vi "SP Save Formatting.vi"(4 "s parameter formatting":T1 {"Plots"."Ch 2"."Reference" format="%#.2g"; "Plots"."Ch 2"."Display Data" items=["Data", "Memory", "Data/Memory"]; "Plots"."Ch 2"."Format" items=["Log Mag", "Phase", "Expanded Phase", "Delay", "Smith", "Polar", "Lin Mag", "SWR", "Loss", "Real", "Imaginary"]; "Plots"."Ch 2"."Scale" min=0.001 step=1.0 format="%#.2g"; "Plots"."Ch 2"."Position" min=0.0 max=10.0; "Plots"."Ch 1"."Reference" format="%#.2g"; "Plots"."Ch 1"."Display Data" items=["Data", "Memory", "Data/Memory"]; "Plots"."Ch 1"."Format" items=["Log Mag", "Phase", "Expanded Phase", "Delay", "Smith", "Polar", "Lin Mag", "SWR", "Loss", "Real", "Imaginary"]; "Plots"."Ch 1"."Scale" min=0.001 step=1.0 format="%#.2g"; "Plots"."Ch 1"."Position" min=0.0 max=10.0}, 5 "error in (no error)":errorcluster, 6 "Cachefile Path (empty)":path, 7 "Object Hierarchy (empty)":string[](array[string]), 8 "tdms file Ref":refnum<k34>) -> (0 "error out":errorcluster, 2 "new Object Hierarchy":string[](array[string]), 3 "dup tdms file Ref":refnum<k34>)   [LabVIEW 2011]
uses:
  server/dd/lib/Report Templates/Template TDM/enumObjectTypes.ctl
  server/dd/lib/Report Templates/Template TDM/enumColor.ctl
  server/dd/lib/Report Templates/Template TDM/enumQueryResultTypes.ctl
  server/dd/lib/Report Templates/Template TDM/enumConditionType.ctl
  server/dd/lib/Report Templates/Template TDM/enumConditionOperator.ctl
  server/dd/lib/Report Templates/Template TDM/objQuery.ctl
  server/dd/lib/Report Templates/Template TDM/enumQueryKeyClass.ctl
  server/dd/lib/Report Templates/Template TDM/enumLineTypes.ctl
  server/dd/lib/Report Templates/Template TDM/enumLineWidths.ctl
  server/dd/lib/Report Templates/Template TDM/enumMarkerTypes.ctl
  TypeDefs/SP Trace.ctl
  TypeDefs/SP Trace Types.ctl
  TypeDefs/SP Frequency Units.ctl
  server/dd/lib/Report Templates/Template TDM/objPlacement.ctl
  TypeDefs/SP Trace Orientation.ctl
  server/dd/lib/Report Templates/Template TDM/enumSummaryOperator.ctl
  TypeDefs/SP Plot Channel.ctl
  TypeDefs/SP Plot Orientation.ctl
  TypeDefs/SP Plot.ctl
  TypeDefs/SP Display Format.ctl
  TypeDefs/SP Display Data.ctl
  TypeDefs/SP Display Trace Controls.ctl
  TypeDefs/SP Formatting.ctl
panel:
  # "Div"
  # "Div"
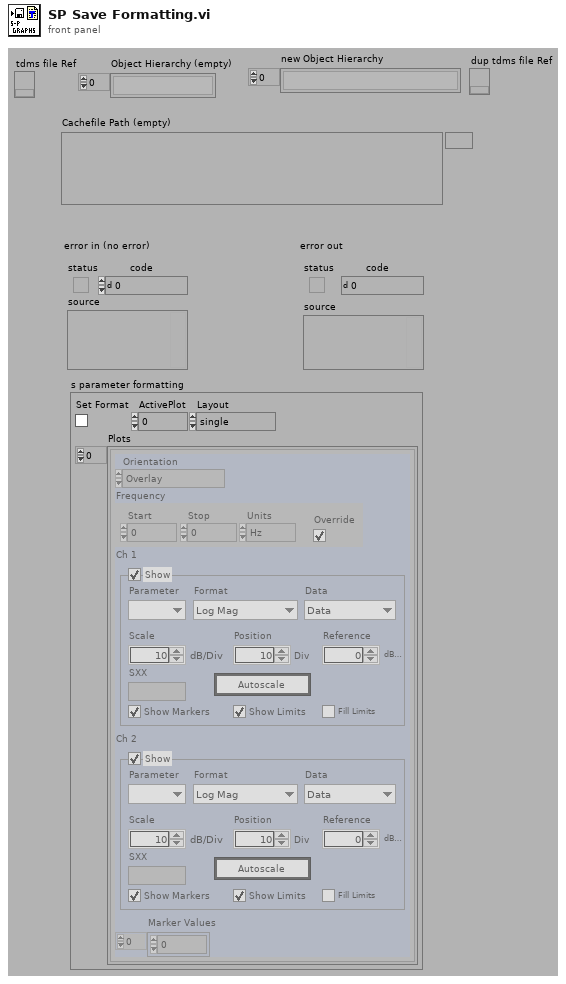
[diagram p1: front panel]
types:
  T1 = typedef "SP Formatting.ctl" = cluster{"Set Format":bool, "Layout":T2, "ActivePlot":i32, "Plots":T3[]}
  T2 = typedef "SP Plot Orientation.ctl" = enum32{"single", "dual", "quad"}
  T3 = typedef "SP Plot.ctl" = cluster{"Orientation":T4, "Ch 1":T5, "Ch 2":T5, "Frequency":cluster{"Start":dbl, "Stop":dbl, "Units":T8, "Override":bool}, "Marker Values":dbl[]}
  T4 = typedef "SP Trace Orientation.ctl" = enum32{"Overlay", "Split"}
  T5 = typedef "SP Display Trace Controls.ctl" = cluster{"Trace On":bool, "Measure":i32, "Format":T6, "Autoscale":bool, "Reference":dbl, "\nRefUnit":string, "Position":dbl, "Scale":dbl, "ScaleUnit":string, "LimitOn":bool, "LimitFill":bool, "Display Data":T7, "Show Markers":bool, "SXX":string}
  T6 = typedef "SP Display Format.ctl" = i32
  T7 = typedef "SP Display Data.ctl" = u16
  T8 = typedef "SP Frequency Units.ctl" = enum16{"Hz", "kHz", "MHz", "GHz", "Points"}
  T9 = enum16{"open", "open or create", "create or replace", "create", "open (read-only)"}
  T10 = typedef "objPlacement.ctl" = cluster{"XPos":dbl, "YPos":dbl, "Width":dbl, "Height":dbl}
  T11 = typedef "enumObjectTypes.ctl" = enum16{"container", "graphics", "text", "picture", "qobject", "sparameterplot", "sparametertrace"}
  T12 = typedef "objQuery.ctl" = cluster{"ResultType":T13, "KeyName":string, "KeyClass":T14, "NoResults":string, "IncludeUnit":bool, "ResultOffset":i32, "SummaryChannel":string, "SummaryFormat":string, "SummaryOperator":T15, "SummaryLimit":i32, "Conditions":cluster{"Type":T16, "Property":string, "Operator":T17, "Value":string}[]}
  T13 = typedef "enumQueryResultTypes.ctl" = enum16{"PropertyValue", "Scalar", "Vector", "Summary"}
  T14 = typedef "enumQueryKeyClass.ctl" = enum16{"File", "Run", "Channel"}
  T15 = typedef "enumSummaryOperator.ctl" = enum16{"avg", "min", "max", "rng", "sum"}
  T16 = typedef "enumConditionType.ctl" = enum16{"eSearchFile", "eSearchChannelGroup", "eSearchChannel"}
  T17 = typedef "enumConditionOperator.ctl" = enum16{"="}
  T18 = typedef "SP Plot Channel.ctl" = cluster{"ChIndex":i32, "Sxx":string, "Format":string, "Autoscale":bool, "Scale":dbl, "RefValue":dbl, "RefPos":dbl, "Fstart":dbl, "Fstop":dbl, "Funit":T8, "Color":T19, "DataQuery":string, "Markers":bool}
  T19 = typedef "enumColor.ctl" = enum16{"black", "red", "green", "blue", "violet", "turquoise", "grey", "yell", "dark red", "dark green", "dark blue", "dark violet", "dark turquoise", "dark grey", "dark yellow", "white", "other colors", "no color"}
  T20 = typedef "SP Trace.ctl" = cluster{"PlotName":string, "TraceSxx":string, "TraceType":T21, "Class":string, "Color":T19, "LineType":T22, "LineWidth":T23, "MarkerType":T24, "MarkerColor":T19, "MarkerSize":dbl}
  T21 = typedef "SP Trace Types.ctl" = enum16{"hidden", "data", "upper limit", "lower limit", "failures", "memory"}
  T22 = typedef "enumLineTypes.ctl" = enum16{"solid", "dash&dott", "dashed 1", "dashed 2", "dotted"}
  T23 = typedef "enumLineWidths.ctl" = enum16{"min", "0.25", "0.35", "0.5", "0.7", "1.0", "1.4", "2.0", "2.8", "4.0", "5.6", "8.0", "11.2", "16.0", "22.4", "32.0"}
  T24 = typedef "enumMarkerTypes.ctl" = enum16{"none", "square", "rhomb", "triangle", "cross", "asterisk", "short dash", "long dash", "plus", "circle"}
  T25 = cluster{"Start":dbl, "Stop":dbl, "Units":T8, "Override":bool}
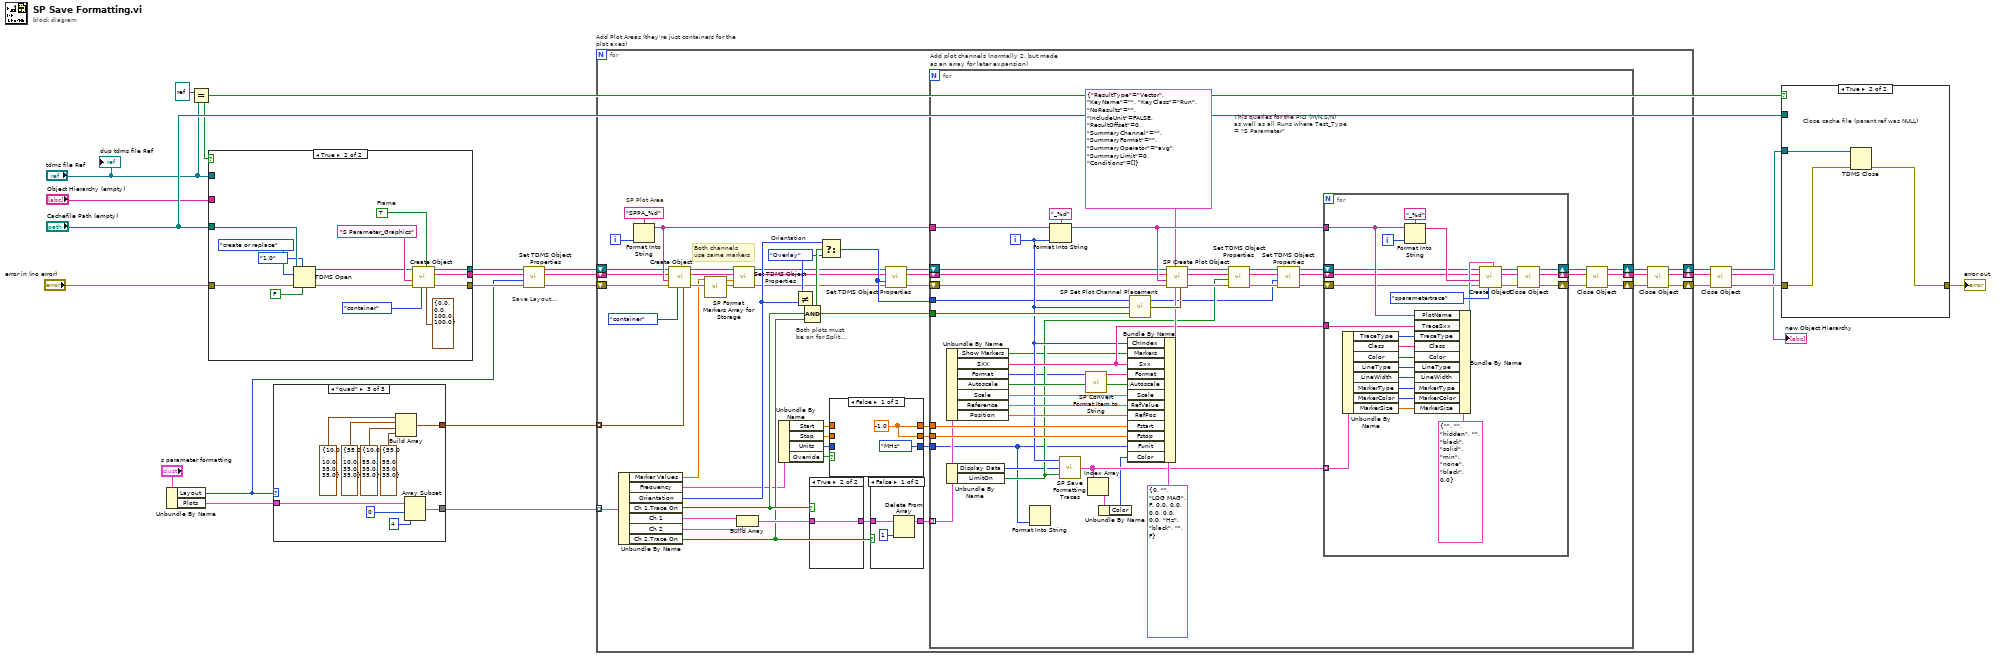
[diagram p0: block diagram]
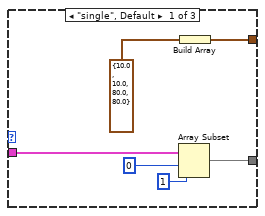
[diagram p2: hidden frame]
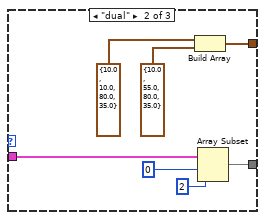
[diagram p3: hidden frame]
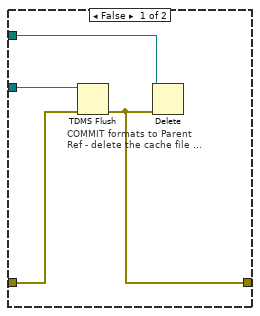
[diagram p4: hidden frame]
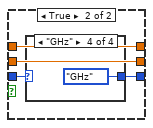
[diagram p6: hidden frame]
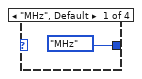
[diagram p7: hidden frame]
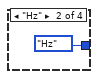
[diagram p8: hidden frame]
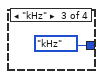
[diagram p9: hidden frame]
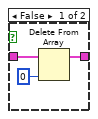
[diagram p11: hidden frame]
diagram:
  # "Save Layout..."
  n1 = Unbundle By Name("s parameter formatting") -> ("Layout"=w17:T2, "Plots"=w22:T3[])
  n2 = Equal?(x=refnum<k34> refnum ("tdms file Ref"), y="tdms file Ref") -> (x = y?=w3:bool)
  n3 = case shown="True" w3 {
    tunnel: "error in (no error)" -> [w27 w36]
    tunnel: "tdms file Ref" -> [w26 _]
    tunnel: [w27 w37] -> w20
    tunnel: "Cachefile Path (empty)" -> [_ w34]
    tunnel: [w25 w31] -> w14
    tunnel: [w26 w30] -> w16
    tunnel: "Object Hierarchy (empty)" -> [w25 _]
    frame False {
    }
    frame True {
      w39 = TRUE  # Frame
      n4 = TDMS Open(6:FALSE ("disable buffering (T)"), 7:enum16{"1.0", "2.0"}."1.0" ("file format version (2.0)"), 8:w36, 10:T9."create or replace" ("operation (0:open)"), 11:w34) -> (0:w35:errorcluster, 3:w32:refnum<k34>)  [unwired: 1 in]
      n5 = call "Create Object.vi"("Object Placement"=T10 {"XPos"=0.0, "YPos"=0.0, "Width"=100.0, "Height"=100.0} ("Placement"), "Properties"=w39, "Object Type (container)"=enumObjectTypes."container", "error in (no error)"=w35, "Object Name (\"\")"="S Parameter_Graphics", "tdms file Ref"=w32) -> ("error out"=w37:errorcluster, "new Object Hierarchy"=w31:string[], "dup tdms file Ref"=w30:refnum<k34>)  [unwired: 2 in, 1 out]
    }
  }
  n6 = case shown="\"quad\"" w17 {
    tunnel: [w46 w52 w62] -> w21
    tunnel: w22 -> [w45 w49 w58]
    tunnel: [w42 w48 w57] -> w1
    frame "single", Default {
      n7 = Array Subset(array=w45, index=0, length=1) -> (w42:T3[])
      n8 = Build Array(T10 {"XPos"=10.0, "YPos"=10.0, "Width"=80.0, "Height"=80.0} ("Placement")) -> (w46:T10[])
    }
    frame "dual" {
      n9 = Build Array(T10 {"XPos"=10.0, "YPos"=10.0, "Width"=80.0, "Height"=35.0} ("Placement"), T10 {"XPos"=10.0, "YPos"=55.0, "Width"=80.0, "Height"=35.0} ("Placement")) -> (w52:T10[])
      n10 = Array Subset(array=w49, index=0, length=2) -> (w48:T3[])
    }
    frame "quad" {
      n11 = Build Array(T10 {"XPos"=10.0, "YPos"=10.0, "Width"=35.0, "Height"=35.0} ("Placement"), T10 {"XPos"=55.0, "YPos"=10.0, "Width"=35.0, "Height"=35.0} ("Placement"), T10 {"XPos"=10.0, "YPos"=55.0, "Width"=35.0, "Height"=35.0} ("Placement"), T10 {"XPos"=55.0, "YPos"=55.0, "Width"=35.0, "Height"=35.0} ("Placement")) -> (w62:T10[])
      n12 = Array Subset(array=w58, index=0, length=4) -> (w57:T3[])
    }
  }
  n13 = call "Set TDMS Object Properties.vi"("error in (no error)"=w20, "Cluster or Control"=w17, "Object Hierarchy (empty)"=w14, "tdms file Ref"=w16) -> ("error out"=w7:errorcluster, "dup Object Hierarchy"=w13:string[], "dup tdms file Ref"=w8:refnum<k34>)  [unwired: 1 out]
  n14 = for "Add Plot Areas (they're just containers for the plot axes)" {
    tunnel: w21 -> [w105] mode=indexing
    tunnel: w1 -> [w104] mode=indexing
    shift-right: [w84] -> w10
    shift-left: w13 -> [w82]
    shift-right: [w78] -> w5
    shift-left: w8 -> [w80]
    shift-right: [w79] -> w6
    shift-left: w7 -> [w81]
    i -> [w107]
    w88 = SP_Trace_Orientation."Overlay"  # Orientation
    # "Both channels\nuse same markers"
    # "Both plots must\nbe on for Split..."
    # "SP Plot Area"
    n15 = Unbundle By Name(w104) -> ("Marker Values"=w66:dbl[], "Frequency"=w87:T25, "Orientation"=w89:T4, "Ch 1.Trace On"=w93:bool, "Ch 1"=w65:T5, "Ch 2"=w64:T5, "Ch 2.Trace On"=w92:bool)
    n16 = Format Into String(format string="SPPA_%d", w107) -> (resulting string=w106:string)  [unwired: 2 in, 1 out]
    n17 = call "Create Object.vi"("Object Placement"=w105, "Object Type (container)"=enumObjectTypes."container", "error in (no error)"=w81, "Object Name (\"\")"=w106, "Object Hierarchy (empty)"=w82, "tdms file Ref"=w80) -> ("error out"=w71:errorcluster, "new Object Hierarchy"=w72:string[], "dup tdms file Ref"=w73:refnum<k34>)  [unwired: 2 in, 1 out]
    n18 = call "SP Format Markers Array for Storage.vi"("Marker Values (none)"=w66) -> ("Marker"=w67:dbl[])  [unwired: 6 out]
    n19 = call "Set TDMS Object Properties.vi"("error in (no error)"=w71, "Cluster or Control"=w67, "Object Hierarchy (empty)"=w72, "tdms file Ref"=w73) -> ("error out"=w68:errorcluster, "dup Object Hierarchy"=w69:string[], "dup tdms file Ref"=w70:refnum<k34>)  [unwired: 1 out]
    n20 = Build Array(w65, w64) -> (w103:T5[])
    n21 = Unbundle By Name(w87) -> ("Start"=w98:dbl, "Stop"=w97:dbl, "Units"=w101:T8, "Override"=w99:bool)
    n22 = Not Equal?(x=w88, y=w89) -> (x != y?=w94:bool)
    n23 = Compound Arithmetic op=AND(w94, w93, w92) -> (w90:bool)
    n24 = case shown="True" w93 {
      tunnel: w103 -> [w126 w127]
      tunnel: [w125 w127] -> w102
      frame False {
        n25 = Delete From Array(array=w126, index=0) -> (array with subset deleted=w125:T5[])  [unwired: 1 in, 1 out]
      }
      frame True {
      }
    }
    n26 = Select(t=w89, s=w90, f=w88) -> (s? t:f=w86:T4)
    n27 = case shown="False" w99 {
      tunnel: w101 -> [_ w115]
      tunnel: [SP_Frequency_Units."MHz" ("Funit") w114] -> w100
      tunnel: w98 -> [_ w112]
      tunnel: w97 -> [_ w113]
      tunnel: [w110 w113] -> w95
      tunnel: [w110 w112] -> w96
      frame False {
        w110 = -1.0 ("Start Frequency")
      }
      frame True {
        n28 = case shown="\"GHz\"" w115 {
          tunnel: [SP_Frequency_Units."MHz" ("Funit") SP_Frequency_Units."Hz" ("Funit") SP_Frequency_Units."kHz" ("Funit") SP_Frequency_Units."GHz" ("Funit")] -> w114
          frame "MHz", Default {
          }
          frame "Hz" {
          }
          frame "kHz" {
          }
          frame "GHz" {
          }
        }
      }
    }
    n29 = case shown="False" w92 {
      tunnel: w102 -> [w122 w123]
      tunnel: [w121 w123] -> w91
      frame False {
        n30 = Delete From Array(array=w122, index=1) -> (array with subset deleted=w121:T5[])  [unwired: 1 in, 1 out]
      }
      frame True {
      }
    }
    n31 = call "Set TDMS Object Properties.vi"("error in (no error)"=w68, "Cluster or Control"=w86, "Object Hierarchy (empty)"=w69, "tdms file Ref"=w70) -> ("error out"=w76:errorcluster, "dup Object Hierarchy"=w85:string[], "dup tdms file Ref"=w77:refnum<k34>)  [unwired: 1 out]
    n32 = for "Add plot channels (normally 2, but made\nas an array for later expansion)" {
      tunnel: w106 -> [w171]
      tunnel: w90 -> [w169]
      tunnel: w91 -> [w159] mode=indexing
      tunnel: w100 -> [w130]
      tunnel: w96 -> [w164]
      tunnel: w95 -> [w165]
      tunnel: w86 -> [w148]
      shift-right: [w143] -> w83
      shift-left: w85 -> [w142]
      shift-right: [w139] -> w74
      shift-left: w77 -> [w140]
      shift-right: [w138] -> w75
      shift-left: w76 -> [w141]
      i -> [w157]
      # "This queries for the PID (M/N,S/N)\nas well as all Runs where Test_Type\n= \"S Parameter\""
      n33 = Unbundle By Name(w159) -> ("Show Markers"=w133:bool, "SXX"=w163:string, "Format"=w129:T6, "Autoscale"=w158:bool, "Scale"=w162:dbl, "Reference"=w161:dbl, "Position"=w160:dbl)
      n34 = Unbundle By Name(w159) -> ("Display Data"=w131:T7, "LimitOn"=w150:bool)
      n35 = Format Into String(w130) -> ()  [unwired: 3 in, 2 out]
      n36 = Format Into String(format string="_%d", initial string=w171, w157) -> (resulting string=w166:string)  [unwired: 1 in, 1 out]
      n37 = call "SP Save Formatting Traces.vi"("LimitOn"=w150, "Display"=w131, "Ch Index (0)"=w157) -> ("Traces"=w155:T20[])
      n38 = call "SP Convert Format Item to String.vi"("Format"=w129) -> ("Format String"=w128:string)  [unwired: 6 out]
      n39 = Index Array(array=w155) -> (element=w154:T20)  [unwired: 1 in]
      n40 = Unbundle By Name(w154) -> ("Color"=w153:T19)
      n41 = Bundle By Name(cluster=T18 {"ChIndex"=0, "Sxx"="", "Format"="LOG MAG", "Autoscale"=FALSE, "Scale"=0.0, "RefValue"=0.0, "RefPos"=0.0, "Fstart"=0.0, "Fstop"=0.0, "Funit"=enum."Hz", "Color"=enum."black", "DataQuery"="", "Markers"=FALSE} ("PlotChannel"), "ChIndex"=w157, "Markers"=w133, "Sxx"=w163, "Format"=w128, "Autoscale"=w158, "Scale"=w162, "RefValue"=w161, "RefPos"=w160, "Fstart"=w164, "Fstop"=w165, "Funit"=w130, "Color"=w153) -> (w167:T18)
      n42 = call "SP Set Plot Channel Placement.vi"("Split? (f = Overlay)"=w169, "ChIndex (0)"=w157) -> ("Placement"=w168:T10)  [unwired: 3 out]
      n43 = call "SP Create Plot Object.vi"("Placement"=w168, "PlotChannel"=w167, "Query"=T12 {"ResultType"=enum."Vector", "KeyName"="", "KeyClass"=enum."Run", "NoResults"="", "IncludeUnit"=FALSE, "ResultOffset"=0, "SummaryChannel"="", "SummaryFormat"="", "SummaryOperator"=enum."avg", "SummaryLimit"=0, "Conditions"=[]} ("objQuery"), "error in (no error)"=w141, "Name"=w166, "Object Hierarchy (empty)"=w142, "tdms file Ref"=w140) -> ("error out"=w156:errorcluster, "new Object Hierarchy"=w146:string[], "dup tdms file Ref"=w152:refnum<k34>)  [unwired: 2 out]
      n44 = call "Set TDMS Object Properties.vi"("error in (no error)"=w156, "Cluster or Control"=w150, "Object Hierarchy (empty)"=w146, "tdms file Ref"=w152) -> ("error out"=w151:errorcluster, "dup Object Hierarchy"=w147:string[], "dup tdms file Ref"=w149:refnum<k34>)  [unwired: 1 out]
      n45 = call "Set TDMS Object Properties.vi"("error in (no error)"=w151, "Cluster or Control"=w148, "Object Hierarchy (empty)"=w147, "tdms file Ref"=w149) -> ("error out"=w136:errorcluster, "dup Object Hierarchy"=w145:string[], "dup tdms file Ref"=w137:refnum<k34>)  [unwired: 1 out]
      n46 = for {
        tunnel: w166 -> [w191]
        tunnel: w163 -> [w192]
        tunnel: w155 -> [w190] mode=indexing
        shift-right: [w179] -> w144
        shift-left: w145 -> [w177]
        shift-right: [w173] -> w134
        shift-left: w136 -> [w175]
        shift-right: [w174] -> w135
        shift-left: w137 -> [w176]
        i -> [w197]
        n47 = Unbundle By Name(w190) -> ("TraceType"=w189:T21, "Class"=w188:string, "Color"=w187:T19, "LineType"=w186:T22, "LineWidth"=w185:T23, "MarkerType"=w184:T24, "MarkerColor"=w183:T19, "MarkerSize"=w182:dbl)
        n48 = Format Into String(format string="_%d", initial string=w191, w197) -> (resulting string=w196:string)  [unwired: 1 in, 1 out]
        n49 = Bundle By Name(cluster=T20 {"PlotName"="", "TraceSxx"="", "TraceType"=enum."hidden", "Class"="", "Color"=enum."black", "LineType"=enum."solid", "LineWidth"=enum."min", "MarkerType"=enum."none", "MarkerColor"=enum."black", "MarkerSize"=0.0} ("Traces"), "PlotName"=w191, "TraceSxx"=w192, "TraceType"=w189, "Class"=w188, "Color"=w187, "LineType"=w186, "LineWidth"=w185, "MarkerType"=w184, "MarkerColor"=w183, "MarkerSize"=w182) -> (w193:T20)
        n50 = call "Create Object.vi"("Properties"=w193, "Object Type (container)"=enumObjectTypes."sparametertrace", "error in (no error)"=w175, "Object Name (\"\")"=w196, "Object Hierarchy (empty)"=w177, "tdms file Ref"=w176) -> ("error out"=w180:errorcluster, "new Object Hierarchy"=w178:string[], "dup tdms file Ref"=w181:refnum<k34>)  [unwired: 2 in, 1 out]
        n51 = call "Close Object.vi"("error in (no error)"=w180, "Object Hierarchy (empty)"=w178, "tdms file Ref"=w181) -> ("error out"=w173:errorcluster, "new Object Hierarchy"=w179:string[], "dup tdms file Ref"=w174:refnum<k34>)  [unwired: 2 out]
      }
      n52 = call "Close Object.vi"("error in (no error)"=w134, "Object Hierarchy (empty)"=w144, "tdms file Ref"=w135) -> ("error out"=w138:errorcluster, "new Object Hierarchy"=w143:string[], "dup tdms file Ref"=w139:refnum<k34>)  [unwired: 2 out]
    }
    n53 = call "Close Object.vi"("error in (no error)"=w75, "Object Hierarchy (empty)"=w83, "tdms file Ref"=w74) -> ("error out"=w79:errorcluster, "new Object Hierarchy"=w84:string[], "dup tdms file Ref"=w78:refnum<k34>)  [unwired: 2 out]
  }
  n54 = call "Close Object.vi"("error in (no error)"=w6, "Object Hierarchy (empty)"=w10, "tdms file Ref"=w5) -> ("error out"=w12:errorcluster, "new Object Hierarchy"=→"new Object Hierarchy":string[], "dup tdms file Ref"=w11:refnum<k34>)  [unwired: 2 out]
  n55 = case shown="True" w3 {
    tunnel: w12 -> [w200 w204]
    tunnel: w11 -> [w201 w205]
    tunnel: [w199 w203] -> w18
    tunnel: "Cachefile Path (empty)" -> [w202 _]
    frame False {
      # "COMMIT formats to Parent\nRef - delete the cache file ..."
      n56 = TDMS Flush(4:w200, 7:w201) -> (0:w199:errorcluster)  [unwired: 1 out]
      n57 = Delete(path (use dialog)=w202, error in=w199) -> ()  [unwired: 6 out]
    }
    frame True {
      # "Close cache file (parent ref was NULL)"
      n58 = TDMS Close(8:w204, 11:w205) -> (0:w203:errorcluster)  [unwired: 1 out]
    }
  }
  "error out" <- w18
  "dup tdms file Ref" <- "tdms file Ref"
